vi "Tab Control - Label--Const.vi"() -> (3 "Tab Control Label":string)   [LabVIEW 2017, in "DTacq Plot Display Library.lvlib"]
uses:
  DTacq Plot Display Library.lvlib
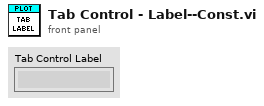
[diagram p1: front panel]
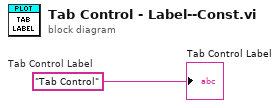
[diagram p0: block diagram]
diagram:
  w1 = "Tab Control"  # Tab Control Label
  "Tab Control Label" <- w1
